vi "NumatoRelay.Set Relay - OLD.vi"(8 "error in":errorcluster, 9 "State":bool, 10 "Relay":i32 min=0 max=7 step=1, 11 "VISA Alias":refnum<visa-resource-name>) -> (0 "error out":errorcluster, 1 "Response":string, 2 "Query":string, 3 "Write":string)   [LabVIEW 2018]
uses:
  <vilib>/Instr/_visa.llb/VISA Configure Serial Port (Instr).vi
  <vilib>/KATE/Time/Time Utils.lvlib
panel:
  out "read 2":string
  out "read 1":string
  in  "Wait(ms)":u32=10
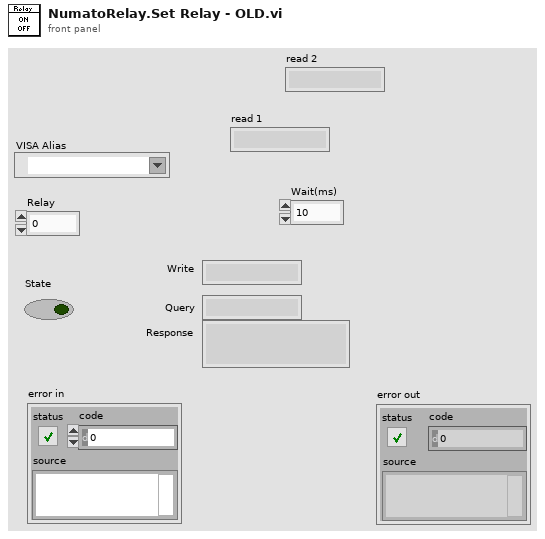
[diagram p1: front panel]
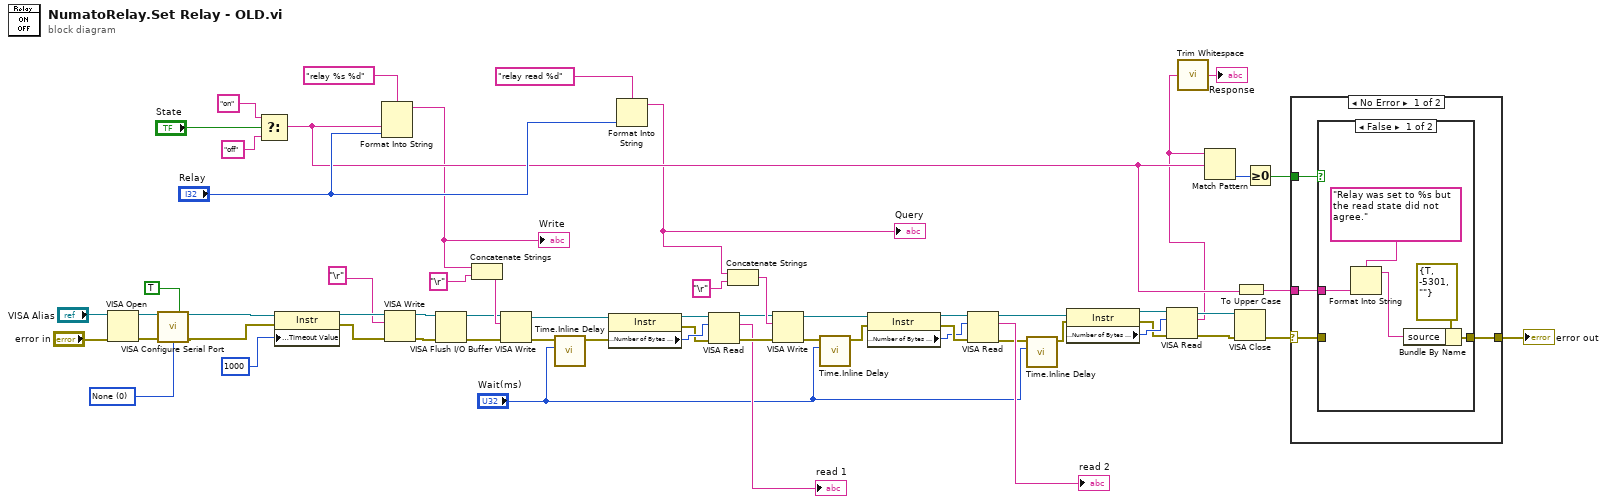
[diagram p0: block diagram]
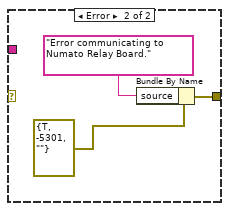
[diagram p3: hidden frame]
diagram:
  w37 = u16 0 items=["None", "XON/XOFF", "RTS/CTS", "XON/XOFF & RTS/CTS", "DTR/DSR", "XON/XOFF & DTR/DSR"] ("flow control (0:none)")
  n1 = VISA Open(error in (no error)="error in", VISA resource name="VISA Alias") -> (VISA resource name=w39:refnum<visa-resource-name>, error out=w38:errorcluster)  [unwired: 3 in]
  n2 = call-poly "VISA Configure Serial Port"("VISA resource name"=w39, "Enable Termination\nChar (T)"=TRUE ("Enable Termination\nChar (T)"), "error in (no error)"=w38, "flow control (0:none)"=w37) -> ("VISA resource name out"=w6:refnum<visa-resource-name>, "error out"=w5:errorcluster)  [unwired: 10 in]
  n3 = Select(t="on", s="State", f="off") -> (s? t:f=w41:string)
  n4 = property class="Instr"(reference=w6, error in=w5, "General Settings:Timeout Value"=u32 1000) -> (reference out=w14:refnum<visa-resource-name>, error out=w13:errorcluster)
  n5 = Format Into String(format string="relay %s %d", w41, "Relay") -> (resulting string=w36:string)  [unwired: 2 in, 1 out]
  "Write" <- w36
  n6 = VISA Write(VISA resource name=w14, write buffer="\r", error in (no error)=w13) -> (VISA resource name out=w12:refnum<visa-resource-name>, error out=w11:errorcluster)  [unwired: 1 out]
  n7 = VISA Flush I/O Buffer(VISA resource name=w12, error in (no error)=w11) -> (VISA resource name out=w9:refnum<visa-resource-name>, error out=w10:errorcluster)  [unwired: 1 in]
  n8 = Concatenate Strings(w36, "\r") -> (w35:string)
  n9 = VISA Write(VISA resource name=w9, write buffer=w35, error in (no error)=w10) -> (VISA resource name out=w29:refnum<visa-resource-name>, error out=w54:errorcluster)  [unwired: 1 out]
  n10 = call <vilib>:"Time.Inline Delay.vi"("Wait(ms)"="Wait(ms)", "error in top"=w54) -> ("error out top"=w28:errorcluster)  [unwired: 8 in, 1 out]
  n11 = property class="Instr"(reference=w29, error in=w28) -> (reference out=w30:refnum<visa-resource-name>, error out=w31:errorcluster, "Serial Settings:Number of Bytes at Serial Port"=w32:u32)
  n12 = Format Into String(format string="relay read %d", "Relay") -> (resulting string=w34:string)  [unwired: 2 in, 1 out]
  "Query" <- w34
  n13 = VISA Read(VISA resource name=w30, byte count=w32, error in (no error)=w31) -> (VISA resource name out=w27:refnum<visa-resource-name>, read buffer=→"read 1":string, error out=w26:errorcluster)  [unwired: 1 out]
  n14 = Concatenate Strings(w34, "\r") -> (w33:string)
  n15 = VISA Write(VISA resource name=w27, write buffer=w33, error in (no error)=w26) -> (VISA resource name out=w51:refnum<visa-resource-name>, error out=w53:errorcluster)  [unwired: 1 out]
  n16 = call <vilib>:"Time.Inline Delay.vi"("Wait(ms)"="Wait(ms)", "error in top"=w53) -> ("error out top"=w50:errorcluster)  [unwired: 8 in, 1 out]
  n17 = property class="Instr"(reference=w51, error in=w50) -> (reference out=w52:refnum<visa-resource-name>, error out=w49:errorcluster, "Serial Settings:Number of Bytes at Serial Port"=w48:u32)
  n18 = VISA Read(VISA resource name=w52, byte count=w48, error in (no error)=w49) -> (VISA resource name out=w18:refnum<visa-resource-name>, read buffer=→"read 2":string, error out=w19:errorcluster)  [unwired: 1 out]
  n19 = call <vilib>:"Time.Inline Delay.vi"("Wait(ms)"="Wait(ms)", "error in top"=w19) -> ("error out top"=w20:errorcluster)  [unwired: 8 in, 1 out]
  n20 = property class="Instr"(reference=w18, error in=w20) -> (reference out=w21:refnum<visa-resource-name>, error out=w22:errorcluster, "Serial Settings:Number of Bytes at Serial Port"=w23:u32)
  n21 = VISA Read(VISA resource name=w21, byte count=w23, error in (no error)=w22) -> (VISA resource name out=w16:refnum<visa-resource-name>, read buffer=w8:string, error out=w15:errorcluster)  [unwired: 1 out]
  n22 = call <vilib>:"Trim Whitespace.vi"("string"=w8) -> ("trimmed string"=→"Response":string)  [unwired: 1 in]
  n23 = Match Pattern(string=w8, regular expression=w41) -> (offset past match=w55:i32)  [unwired: 1 in, 3 out]
  n24 = VISA Close(VISA resource name=w16, error in (no error)=w15) -> (error out=w44:errorcluster)
  n25 = To Upper Case(1:w41) -> (0:w40:string)
  n26 = Greater Or Equal To 0?(x=w55) -> (x >= 0?=w45:bool)
  n27 = case shown="No Error" w44 {
    selector: w44 -> [w64 _]
    tunnel: w45 -> [w65 _]
    tunnel: [w63 w71] -> w43
    tunnel: w40 -> [w62 _]
    frame No Error {
      n28 = case shown="False" w65 {
        tunnel: w64 -> [_ _]
        tunnel: [w69 _] -> w63
        tunnel: w62 -> [w67 _]
        frame False {
          n29 = Format Into String(format string="Relay was set to %s but the read state did not agree.", w67) -> (resulting string=w66:string)  [unwired: 2 in, 1 out]
          n30 = Bundle By Name(cluster=errorcluster {"status"=TRUE, "code"=-5301, "source"=""} ("error constant"), "source"=w66) -> (w69:errorcluster)
        }
        frame True {
        }
      }
    }
    frame Error {
      n31 = Bundle By Name(cluster=errorcluster {"status"=TRUE, "code"=-5301, "source"=""} ("error constant"), "source"="Error communicating to Numato Relay Board.") -> (w71:errorcluster)
    }
  }
  "error out" <- w43
